vi "SVX Buffer Polar Plot.vi"(0 "polar plot data in":T1(array[cluster]), 1 "buffer mode":u16(ring)=1 items=["Infinite length", "Last block data", "Custom"], 2 "reset? (F)":bool, 7 "buffer size":dbl, 11 "error in (no error)":errorcluster) -> (4 "polar plot data out":T1(array[cluster]), 15 "error out":errorcluster)   [LabVIEW 2017, in "SoundVib_OAVisualization.lvlib"]
doc: "Buffers polar plot data according to different buffer modes. This VI requires continuous input data. The buffered data might have gaps between or overlap with previous buffers. Do not use the buffered data for limit testing or data logging."
uses:
  <vilib>/addons/Sound and Vibration/Order Analysis/Data Presentation/SoundVib_OAVisualization.lvlib
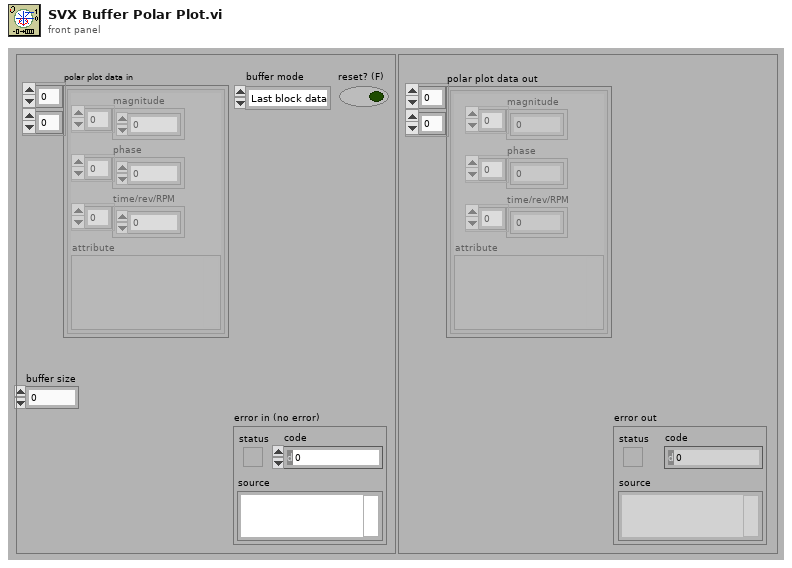
[diagram p1: front panel]
types:
  T1 = cluster{"magnitude":dbl[], "phase":dbl[], "time/rev/RPM":dbl[], "attribute":variant}[][]
  T2 = cluster{"magnitude":dbl[], "phase":dbl[], "time/rev/RPM":dbl[], "attribute":variant}[]
  T3 = cluster{"magnitude":dbl[], "phase":dbl[], "time/rev/RPM":dbl[], "attribute":variant}
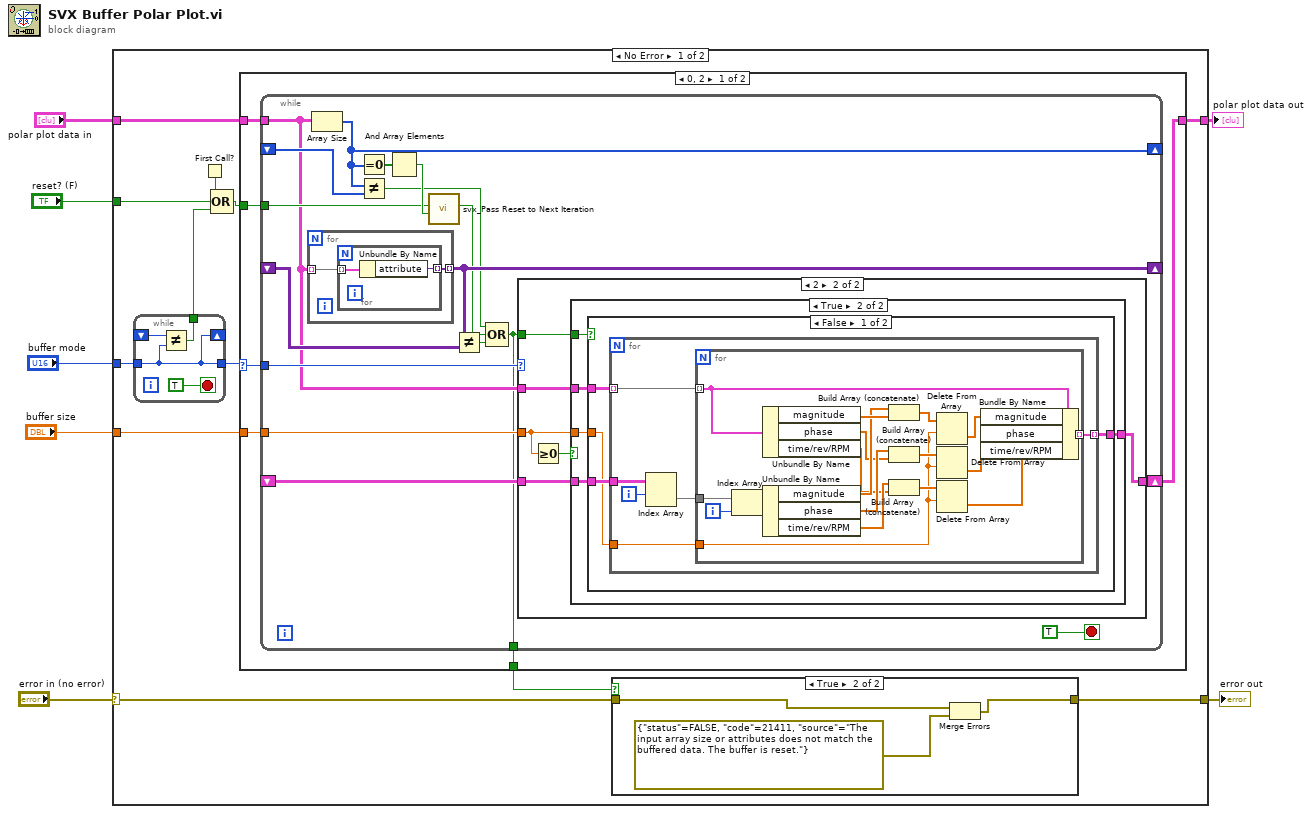
[diagram p0: block diagram]
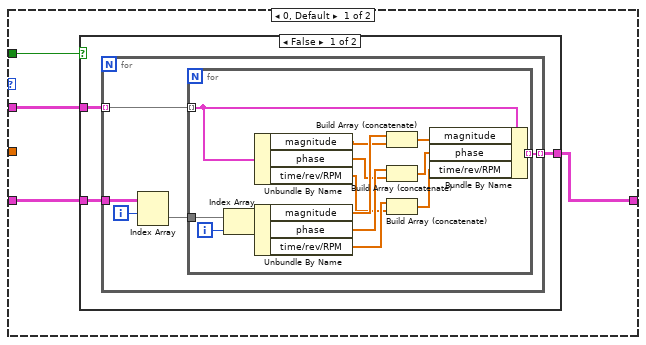
[diagram p3: hidden frame]
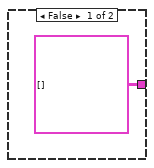
[diagram p5: hidden frame]
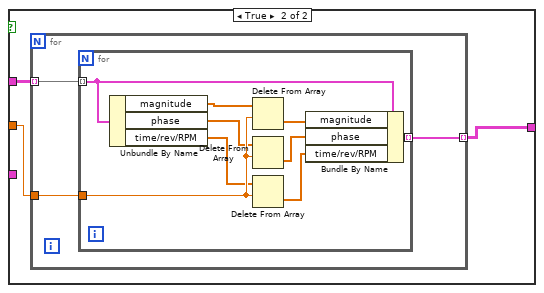
[diagram p6: hidden frame]
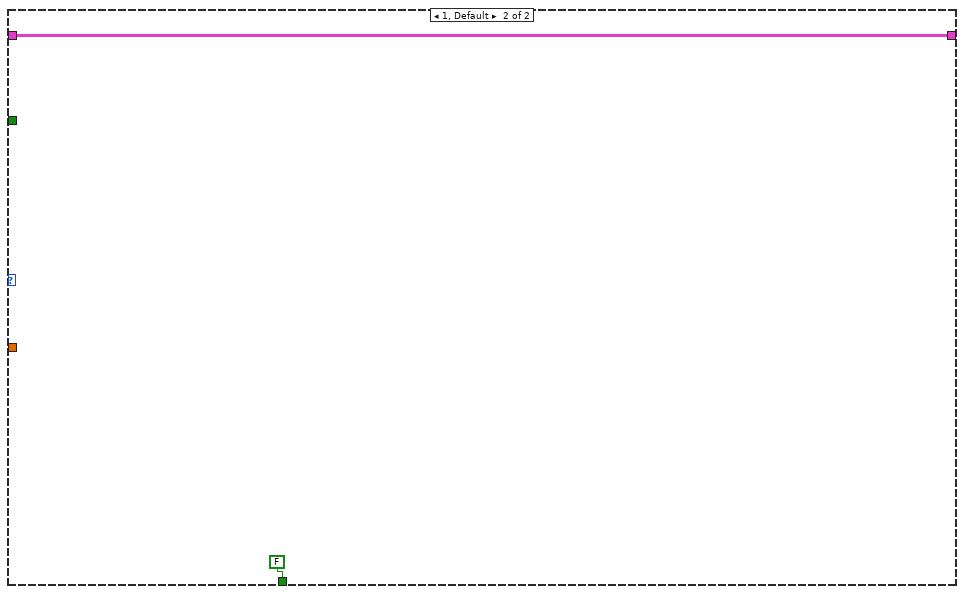
[diagram p7: hidden frame]
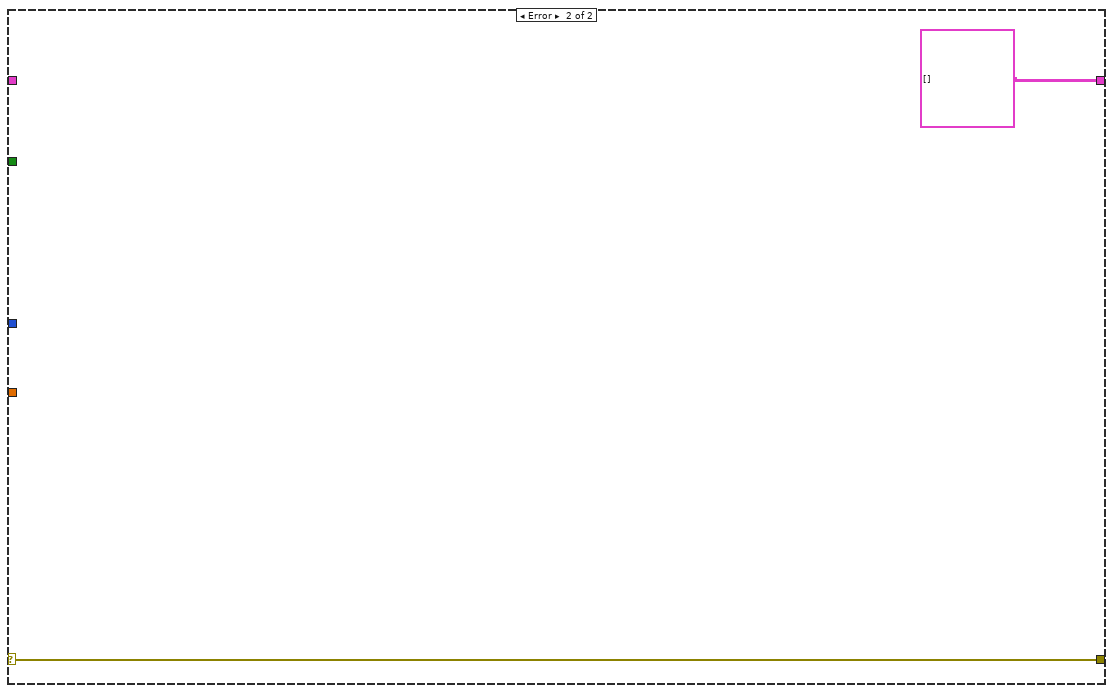
[diagram p8: hidden frame]
diagram:
  n1 = case shown="No Error" "error in (no error)" {
    selector: "error in (no error)" -> [w10 w139]
    tunnel: "polar plot data in" -> [w19 _]
    tunnel: "reset? (F)" -> [w14 _]
    tunnel: "buffer mode" -> [w16 _]
    tunnel: [w18 T1 [] ("polar plot data")] -> w3
    tunnel: [w9 w139] -> w2
    tunnel: "buffer size" -> [w17 _]
    frame No Error {
      n2 = while {
        tunnel: w16 -> [w25]
        tunnel: [w25] -> w15
        shift-right: [w25] -> _
        shift-left: _ -> [w26]
        tunnel: [w24] -> w12
        stop <- TRUE stop-if-true
        n3 = Not Equal?(x=w26, y=w25) -> (x != y?=w24:bool)
      }
      n4 = First Call?() -> (First Call?: T/F=w8:bool)
      n5 = Compound Arithmetic op=OR(w8, w14, w12) -> (w13:bool)
      n6 = case shown="0, 2" w15 {
        selector: w15 -> [w31 _]
        tunnel: w19 -> [w33 w138]
        tunnel: w13 -> [w32 _]
        tunnel: [w29 w138] -> w18
        tunnel: w17 -> [w30 _]
        tunnel: [w28 FALSE] -> w11
        frame 0, 2 {
          n7 = while {
            tunnel: w33 -> [w37]
            shift-right: [w46] -> _
            shift-left: _ -> [w49]
            shift-right: [w47] -> _
            shift-left: _ -> [w48]
            tunnel: w32 -> [w43]
            tunnel: w31 -> [w39]
            tunnel: w30 -> [w38]
            shift-right: [w36] -> w29
            shift-left: _ -> [w35]
            tunnel: [w34] -> w28
            stop <- TRUE stop-if-true
            n8 = for {
              tunnel: w37 -> [w134] mode=indexing
              tunnel: [w133] -> w47 mode=indexing
              n9 = for {
                tunnel: w134 -> [w136] mode=indexing
                tunnel: [w135] -> w133 mode=indexing
                n10 = Unbundle By Name(w136) -> ("attribute"=w135:variant)
              }
            }
            n11 = Array Size(array=w37) -> (size(s)=w46:i32[])
            n12 = Equal To 0?(x=w46) -> (x = 0?=w45:bool[])
            n13 = Not Equal?(x=w46, y=w49) -> (x != y?=w41:bool)
            n14 = And Array Elements(Boolean array=w45) -> (logical AND=w44:bool)
            n15 = call <vilib>:"svx_Pass Reset to Next Iteration.vi"("trigger"=w44, "reset?(F)"=w43) -> ("reset out"=w40:bool)  [unwired: 9 in]
            n16 = Not Equal?(x=w47, y=w48) -> (x != y?=w42:bool)
            n17 = Compound Arithmetic op=OR(w41, w40, w42) -> (w34:bool)
            n18 = case shown="2" w39 {
              tunnel: w38 -> [_ w78]
              tunnel: w34 -> [w54 w81]
              tunnel: w37 -> [w53 w83]
              tunnel: [w52 w80] -> w36
              tunnel: w35 -> [w51 w82]
              frame 0, Default {
                n19 = case shown="False" w54 {
                  tunnel: w53 -> [w57 w77]
                  tunnel: [w55 w77] -> w52
                  tunnel: w51 -> [w56 _]
                  frame False {
                    n20 = for {
                      tunnel: w57 -> [w59] mode=indexing
                      tunnel: w56 -> [w61]
                      tunnel: [w58] -> w55 mode=indexing
                      i -> [w62]
                      n21 = Index Array(array=w61, index (row)=w62) -> (element=w60:T2)  [unwired: 1 in]
                      n22 = for {
                        tunnel: w60 -> [w76]
                        tunnel: w59 -> [w73] mode=indexing
                        tunnel: [w69] -> w58 mode=indexing
                        i -> [w75]
                        n23 = Index Array(array=w76, index=w75) -> (element=w74:T3)
                        n24 = Unbundle By Name(w73) -> ("magnitude"=w67:dbl[], "phase"=w65:dbl[], "time/rev/RPM"=w63:dbl[])
                        n25 = Unbundle By Name(w74) -> ("magnitude"=w68:dbl[], "phase"=w66:dbl[], "time/rev/RPM"=w64:dbl[])
                        n26 = Build Array (concatenate)(w68, w67) -> (w72:dbl[])
                        n27 = Build Array (concatenate)(w66, w65) -> (w71:dbl[])
                        n28 = Build Array (concatenate)(w64, w63) -> (w70:dbl[])
                        n29 = Bundle By Name(cluster=w73, "magnitude"=w72, "phase"=w71, "time/rev/RPM"=w70) -> (w69:T3)
                      }
                    }
                  }
                  frame True {
                  }
                }
              }
              frame 2 {
                n30 = Greater Or Equal To 0?(x=w78) -> (x >= 0?=w79:bool)
                n31 = case shown="True" w79 {
                  tunnel: w83 -> [_ w89]
                  tunnel: w82 -> [_ w88]
                  tunnel: w81 -> [_ w87]
                  tunnel: w78 -> [_ w86]
                  tunnel: [T1 [] w85] -> w80
                  frame False {
                  }
                  frame True {
                    n32 = case shown="False" w87 {
                      tunnel: w89 -> [w93 w120]
                      tunnel: [w91 w118] -> w85
                      tunnel: w88 -> [w92 _]
                      tunnel: w86 -> [w90 w119]
                      frame False {
                        n33 = for {
                          tunnel: w93 -> [w96] mode=indexing
                          tunnel: w92 -> [w98]
                          tunnel: [w95] -> w91 mode=indexing
                          tunnel: w90 -> [w94]
                          i -> [w99]
                          n34 = Index Array(array=w98, index (row)=w99) -> (element=w97:T2)  [unwired: 1 in]
                          n35 = for {
                            tunnel: w97 -> [w117]
                            tunnel: w96 -> [w114] mode=indexing
                            tunnel: [w113] -> w95 mode=indexing
                            tunnel: w94 -> [w109]
                            i -> [w116]
                            n36 = Index Array(array=w117, index=w116) -> (element=w115:T3)
                            n37 = Unbundle By Name(w114) -> ("magnitude"=w105:dbl[], "phase"=w102:dbl[], "time/rev/RPM"=w100:dbl[])
                            n38 = Unbundle By Name(w115) -> ("magnitude"=w104:dbl[], "phase"=w103:dbl[], "time/rev/RPM"=w101:dbl[])
                            n39 = Build Array (concatenate)(w104, w105) -> (w112:dbl[])
                            n40 = Build Array (concatenate)(w103, w102) -> (w111:dbl[])
                            n41 = Build Array (concatenate)(w101, w100) -> (w110:dbl[])
                            n42 = Delete From Array(array=w112, length=w109) -> (deleted portion=w108:dbl[])  [unwired: 1 in, 1 out]
                            n43 = Delete From Array(array=w111, length=w109) -> (deleted portion=w107:dbl[])  [unwired: 1 in, 1 out]
                            n44 = Delete From Array(array=w110, length=w109) -> (deleted portion=w106:dbl[])  [unwired: 1 in, 1 out]
                            n45 = Bundle By Name(cluster=w114, "magnitude"=w108, "phase"=w107, "time/rev/RPM"=w106) -> (w113:T3)
                          }
                        }
                      }
                      frame True {
                        n46 = for {
                          tunnel: w120 -> [w123] mode=indexing
                          tunnel: w119 -> [w122]
                          tunnel: [w121] -> w118 mode=indexing
                          n47 = for {
                            tunnel: w123 -> [w128] mode=indexing
                            tunnel: w122 -> [w131]
                            tunnel: [w124] -> w121 mode=indexing
                            n48 = Unbundle By Name(w128) -> ("magnitude"=w132:dbl[], "phase"=w130:dbl[], "time/rev/RPM"=w129:dbl[])
                            n49 = Delete From Array(array=w132, length=w131) -> (deleted portion=w127:dbl[])  [unwired: 1 in, 1 out]
                            n50 = Delete From Array(array=w130, length=w131) -> (deleted portion=w126:dbl[])  [unwired: 1 in, 1 out]
                            n51 = Delete From Array(array=w129, length=w131) -> (deleted portion=w125:dbl[])  [unwired: 1 in, 1 out]
                            n52 = Bundle By Name(cluster=w128, "magnitude"=w127, "phase"=w126, "time/rev/RPM"=w125) -> (w124:T3)
                          }
                        }
                      }
                    }
                  }
                }
              }
            }
          }
        }
        frame 1, Default {
        }
      }
      n53 = case shown="True" w11 {
        tunnel: w10 -> [w20 w23]
        tunnel: [w20 w22] -> w9
        frame False {
        }
        frame True {
          n54 = Merge Errors(w23, errorcluster {"status"=FALSE, "code"=21411, "source"="The input array size or attributes does not match the buffered data. The buffer is reset."} ("error in 2 (no error)")) -> (w22:errorcluster)
        }
      }
    }
    frame Error {
    }
  }
  "polar plot data out" <- w3
  "error out" <- w2
